vi "CRYSet Signal Generator Front Panel.vi"(11 "Vi Ref in":refnum<vi> caption="Vi Ref") -> (3 "Vi Ref out":refnum<vi> caption="Vi Ref")   [LabVIEW 2013]
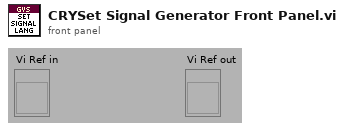
[diagram p1: front panel]
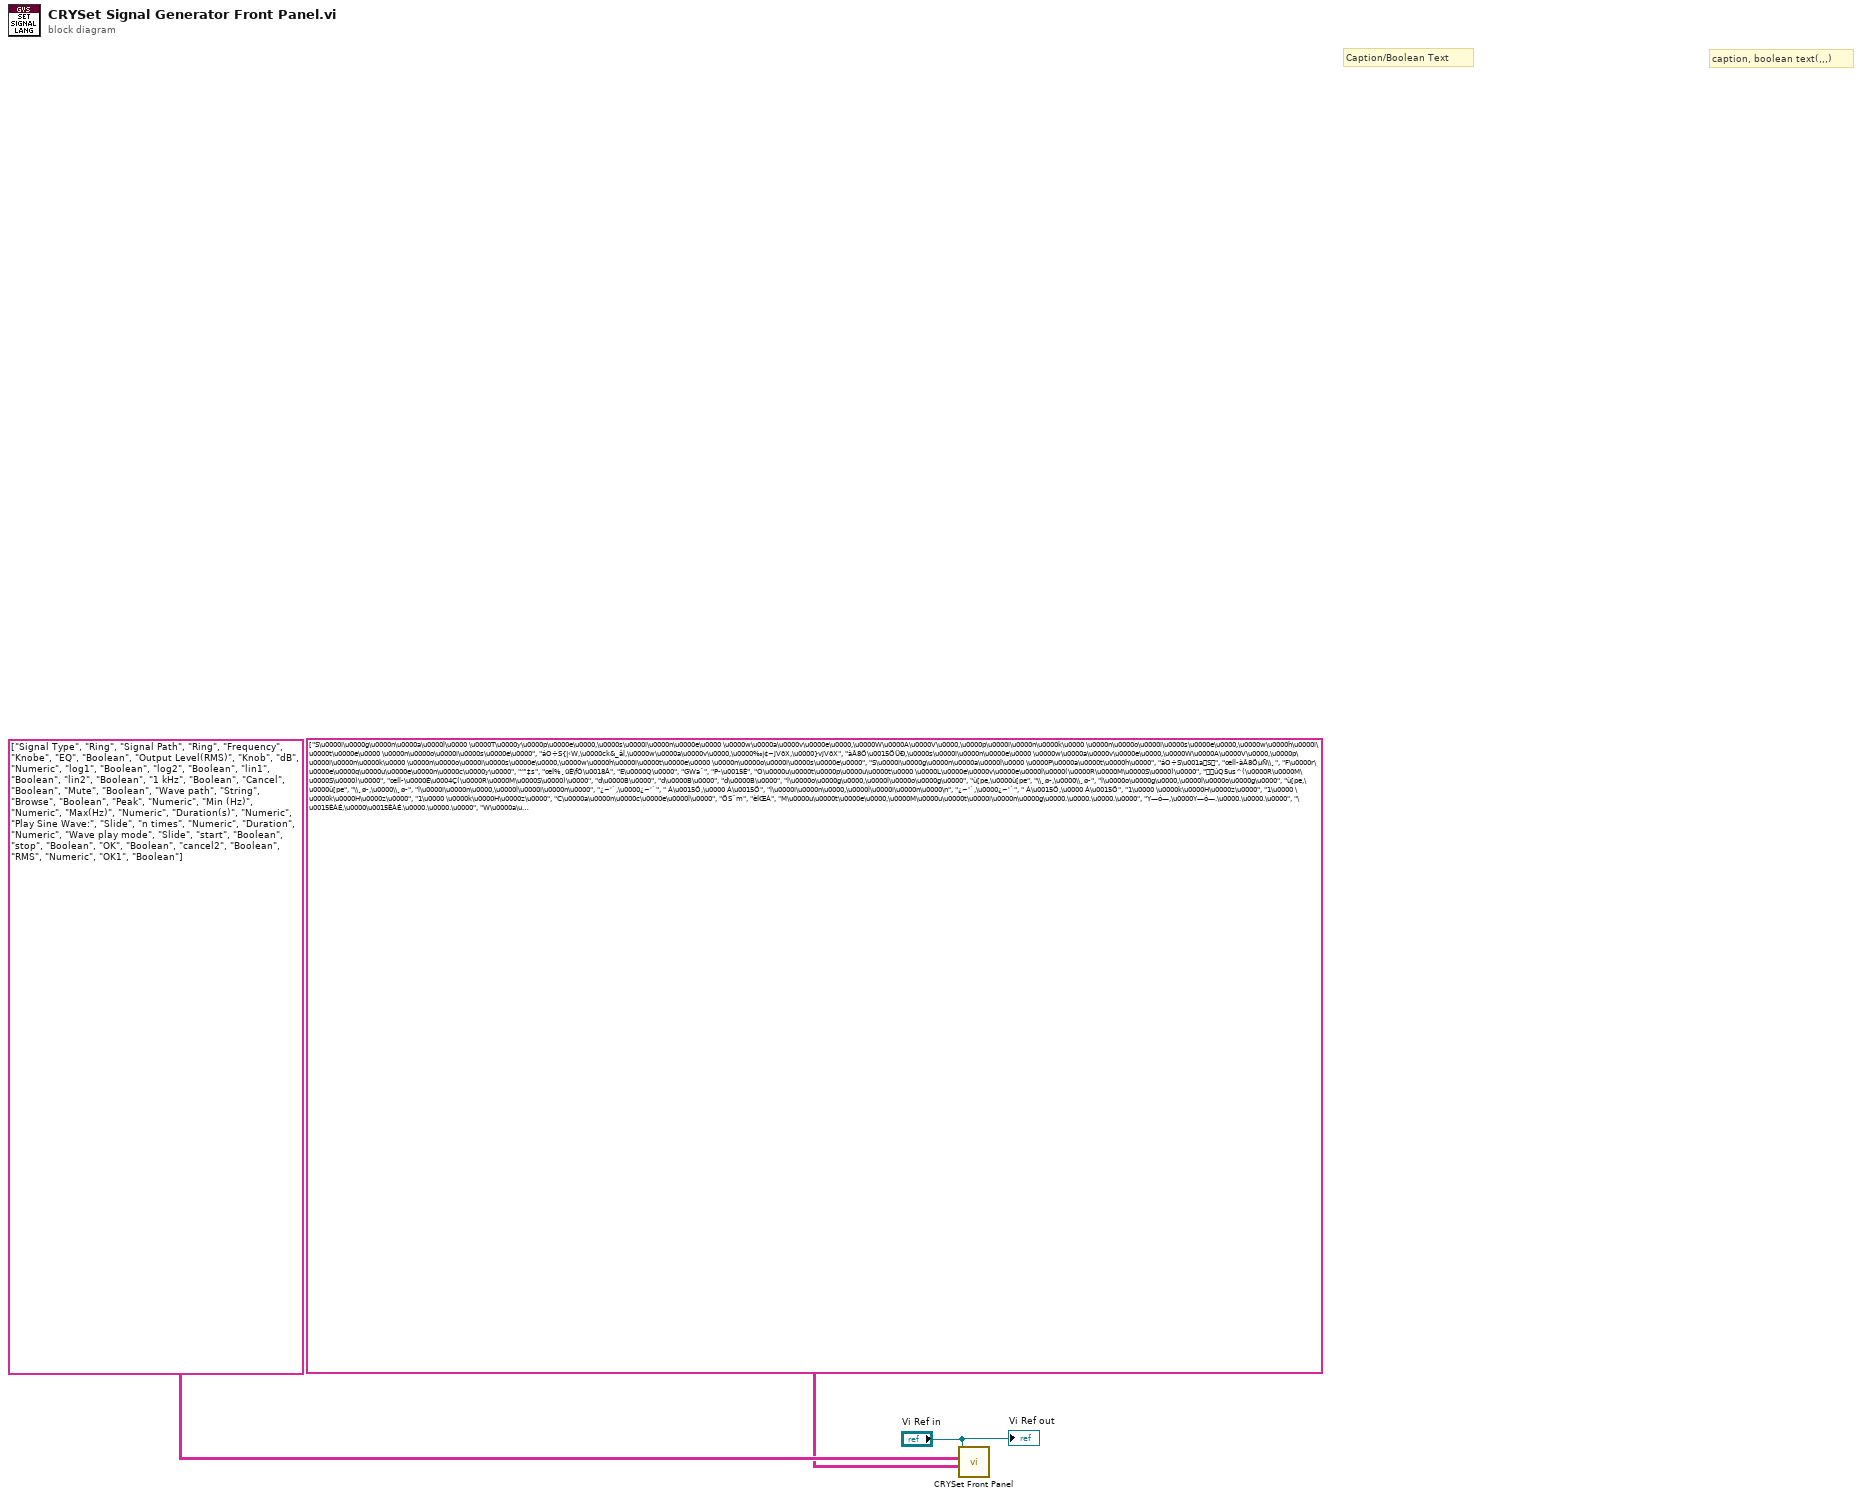
[diagram p0: block diagram]
diagram:
  # "caption, boolean text(,,,)"
  # "Caption/Boolean Text"
  n1 = call "CRYSet Front Panel.vi"("Caption(Boolean Text)"=string[][] [["S\u0000i\u0000g\u0000n\u0000a\u0000l\u0000 \u0000T\u0000y\u0000p\u0000e\u0000,\u0000s\u0000i\u0000n\u0000e\u0000 \u0000w\u0000a\u0000v\u0000e\u0000,\u0000W\u0000A\u0000V\u0000,\u0000p\u0000i\u0000n\u0000k\u0000 \u0000n\u0000o\u0000i\u0000s\u0000e\u0000,\u0000w\u0000h\u0000i\u0000t\u0000e\u0000 \u0000n\u0000o\u0000i\u0000s\u0000e\u0000", "áO÷S{|‹W,\u0000ck&_âl,\u0000w\u0000a\u0000v\u0000,\u0000‰|¢~jVðX,\u0000}vjVðX", "àÂ8Ö\u0015ÖÜÐ,\u0000s\u0000i\u0000n\u0000e\u0000 \u0000w\u0000a\u0000v\u0000e\u0000,\u0000W\u0000A\u0000V\u0000,\u0000p\u0000i\u0000n\u0000k\u0000 \u0000n\u0000o\u0000i\u0000s\u0000e\u0000,\u0000w\u0000h\u0000i\u0000t\u0000e\u0000 \u0000n\u0000o\u0000i\u0000s\u0000e\u0000"], ["S\u0000i\u0000g\u0000n\u0000a\u0000l\u0000 \u0000P\u0000a\u0000t\u0000h\u0000", "áO÷S\u001aS", "œÍl­àÂ8ÖµÑ\\¸"], ["F\u0000r\u0000e\u0000q\u0000u\u0000e\u0000n\u0000c\u0000y\u0000", "‘˜‡s", "œÍ%¸üÈ\fÓ\u0018Â"], ["E\u0000Q\u0000", "GWaˆ", "P­\u0015È"], ["O\u0000u\u0000t\u0000p\u0000u\u0000t\u0000 \u0000L\u0000e\u0000v\u0000e\u0000l\u0000(\u0000R\u0000M\u0000S\u0000)\u0000", "úQ5us^(\u0000R\u0000M\u0000S\u0000)\u0000", "œÍl­\u0000É\u0004Ç(\u0000R\u0000M\u0000S\u0000)\u0000"], ["d\u0000B\u0000", "d\u0000B\u0000", "d\u0000B\u0000"], ["l\u0000o\u0000g\u0000,\u0000l\u0000o\u0000g\u0000", "ù[pe,\u0000ù[pe", "\\¸ø­,\u0000\\¸ø­"], ["l\u0000o\u0000g\u0000,\u0000l\u0000o\u0000g\u0000", "ù[pe,\u0000ù[pe", "\\¸ø­,\u0000\\¸ø­"], ["l\u0000i\u0000n\u0000,\u0000l\u0000i\u0000n\u0000", "¿~'`,\u0000¿~'`", " Á\u0015Ö,\u0000 Á\u0015Ö"], ["l\u0000i\u0000n\u0000,\u0000l\u0000i\u0000n\u0000\n", "¿~'`,\u0000¿~'`", " Á\u0015Ö,\u0000 Á\u0015Ö"], ["1\u0000 \u0000k\u0000H\u0000z\u0000", "1\u0000 \u0000k\u0000H\u0000z\u0000", "1\u0000 \u0000k\u0000H\u0000z\u0000"], ["C\u0000a\u0000n\u0000c\u0000e\u0000l\u0000", "ÖSˆm", "èÍŒÁ"], ["M\u0000u\u0000t\u0000e\u0000,\u0000M\u0000u\u0000t\u0000i\u0000n\u0000g\u0000.\u0000.\u0000.\u0000", "Y—ó—,\u0000Y—ó—.\u0000.\u0000.\u0000", "\u0015ÈÀÉ,\u0000\u0015ÈÀÉ.\u0000.\u0000.\u0000"], ["W\u0000a\u0000v\u0000e\u0000 \u0000F\u0000i\u0000l\u0000e\u0000 \u0000P\u0000a\u0000t\u0000h\u0000", "âleöNï_", "¬ÇÝÀ\fÓ|Ç"], ["B\u0000r\u0000o\u0000w\u0000s\u0000e\u0000.\u0000.\u0000.\u0000", "Omȉ.\u0000.\u0000.\u0000", "ôÅ0®.\u0000.\u0000.\u0000"], ["P\u0000e\u0000a\u0000k\u0000", "\u0000g'Y<P", "\\Í\u0000³\u0012¬"], ["M\u0000i\u0000n\u0000 \u0000(\u0000H\u0000z\u0000)\u0000", "\u0000g\u000f\\(\u0000H\u0000z\u0000)\u0000", "\\ÍŒÁ(\u0000H\u0000z\u0000)\u0000"], ["M\u0000a\u0000x\u0000(\u0000H\u0000z\u0000)\u0000", "\u0000g'Y(\u0000H\u0000z\u0000)\u0000", "\\Í\u0000³(\u0000H\u0000z\u0000)\u0000"], ["D\u0000u\u0000r\u0000a\u0000t\u0000i\u0000o\u0000n\u0000(\u0000s\u0000)\u0000", "öeô•(\u0000Òy)\u0000", "ÜÂ\u0004¬(\u0000\bÍ)\u0000"], ["P\u0000l\u0000a\u0000y\u0000 \u0000S\u0000i\u0000n\u0000e\u0000 \u0000W\u0000a\u0000v\u0000e\u0000:\u0000,\u0000i\u0000n\u0000 \u0000C\u0000o\u0000n\u0000t\u0000i\u0000n\u0000u\u0000o\u0000u\u0000s\u0000 \u0000L\u0000o\u0000o\u0000p\u0000,\u0000f\u0000o\u0000r\u0000 \u0000D\u0000u\u0000r\u0000a\u0000t\u0000i\u0000o\u0000n\u0000", "­d>eck&_áO÷S,\u0000ç~í~,\u0000\u0001cí~öeô•", "¬ÇÝÀ\u0015ÖÜÐ,\u0000(¸Á\u001cÂXÖ,\u0000ÀÉÁÜÂ\u0004¬"], ["N\u0000 \u0000t\u0000i\u0000m\u0000e\u0000s\u0000", "N\u0000!k", "\u0018¼õ¼\u0018Â"], ["s\u0000e\u0000c\u0000", "Òy", "\bÍ"], ["P\u0000l\u0000a\u0000y\u0000 \u0000W\u0000a\u0000v\u0000e\u0000 \u0000F\u0000i\u0000l\u0000e\u0000:\u0000,\u0000,\u0000i\u0000n\u0000 \u0000C\u0000o\u0000n\u0000t\u0000i\u0000n\u0000u\u0000o\u0000u\u0000s\u0000 \u0000L\u0000o\u0000o\u0000p\u0000,\u0000f\u0000o\u0000r\u0000 \u0000D\u0000u\u0000r\u0000a\u0000t\u0000i\u0000o\u0000n\u0000,\u0000N\u0000 \u0000t\u0000i\u0000m\u0000e\u0000s\u0000", "­d>eâl‡eöN,\u0000ç~í~,\u0000\u0001cí~öeô•,\u0000\rP", "¬ÇÝÀ\u0015ÖÜÐ,\u0000(¸Á\u001cÂXÖ,\u0000ÀÉÁÜÂ\u0004¬,\u0000Ö\u0018ÂÀÉ\u0015È"], ["S\u0000t\u0000a\u0000r\u0000t\u0000,\u0000P\u0000l\u0000a\u0000y\u0000i\u0000n\u0000g\u0000.\u0000.\u0000.\u0000", "\u0000_ËY,\u0000­d>e.\u0000.\u0000.\u0000", "ÜÂ‘Ç,\u0000¬ÇÝÀ.\u0000.\u0000.\u0000"], ["S\u0000t\u0000o\u0000p\u0000", "\\Pbk", "\u0015ÈÀÉ"], ["O\u0000K\u0000", "nx¤‹", "UÖxÇ"], ["C\u0000a\u0000n\u0000c\u0000e\u0000l\u0000", "ÖSˆm", "èÍŒÁ"], ["R\u0000M\u0000S\u0000", "R\u0000M\u0000S\u0000", "R\u0000M\u0000S\u0000"], ["O\u0000K\u0000", "nx¤‹", "UÖxÇ"]], "Control ID and Type(Label Name, Type)"=string[][] [["Signal Type", "Ring"], ["Signal Path", "Ring"], ["Frequency", "Knobe"], ["EQ", "Boolean"], ["Output Level(RMS)", "Knob"], ["dB", "Numeric"], ["log1", "Boolean"], ["log2", "Boolean"], ["lin1", "Boolean"], ["lin2", "Boolean"], ["1 kHz", "Boolean"], ["Cancel", "Boolean"], ["Mute", "Boolean"], ["Wave path", "String"], ["Browse", "Boolean"], ["Peak", "Numeric"], ["Min (Hz)", "Numeric"], ["Max(Hz)", "Numeric"], ["Duration(s)", "Numeric"], ["Play Sine Wave:", "Slide"], ["n times", "Numeric"], ["Duration", "Numeric"], ["Wave play mode", "Slide"], ["start", "Boolean"], ["stop", "Boolean"], ["OK", "Boolean"], ["cancel2", "Boolean"], ["RMS", "Numeric"], ["OK1", "Boolean"]], "Vi Ref"="Vi Ref in") -> ()  [unwired: 9 in]
  "Vi Ref out" <- "Vi Ref in"
